vi "CPT32(Host).vi"() -> ()   [LabVIEW 2021]
uses:
  Control 1.ctl
  CPTLOCKIN/Control 2.ctl
  <vilib>/FPGAPlugInAG/PCIe-7857/niLvFpga_Open_PCIe-7857.vi
  <vilib>/rvi/interface/common/dynamic/niFpgaDynamicAddResources.vi
  <vilib>/Utility/error.llb/Error Cluster From Error Code.vi
  <vilib>/rvi/errors/niLvFpgaAdjustHostInterfaceError.vi
  <vilib>/FPGAPlugInAG/Dynamic/niLvFpga_Close_Dynamic.vi
  <vilib>/rvi/interface/nirviOpenFPGA/nirviOpenFPGA.xnode
  FPGA Bitfiles/lvfpga32_FPGATarget_CPT32PulseGen3(F_lvzEpAMTsdg.lvbitx
  FPGA Target/CPT32 Pulse Gen 3 (FPGA).vi
  <vilib>/rvi/interface/nirviReadWriteControl/nirviReadWriteControl.xnode
  <vilib>/rvi/interface/nirviCloseFPGA/nirviCloseFPGA.xnode
  <vilib>/rvi/interface/Simulation/niFpgaSimulationCallBeginRW.vi
  NiFpgaLv.dll
panel:
  in  "Tab Control":enum32{"数字与模拟信号控制"}(tab)
  in  "DO 0-7（ms）":T3={"DO 0"=[10.0, 0.0, 0.0, 0.0, 0.0, 0.0, 0.0, 0.0, 0.0, 0.0, 0.0, 0.0, 0.0, 0.0, 0.0, 0.0], "DO 1"=[-106.0, 0.2998046875, -20.0, 0.009765625, 0.0, 0.0, 0.0, 0.0, 0.0, 0.0, 0.0, 0.0, 0.0, 0.0, 0.0, 0.0, 0.0, 0.0, 0.0, 0.0, 0.0, 0.0, 0.0, 0.0, 0.0, 0.0, 0.0, 0.0, 0.0, 0.0, 0.0, 0.0], "DO 2"=[100.0, 5.0, 0.0, 0.0, 0.0, 0.0, 0.0, 0.0, 0.0, 0.0, 0.0, 0.0, 0.0, 0.0, 0.0, 0.0], "DO 3"=[100.0, 5.0, 0.0, 0.0, 0.0, 0.0, 0.0, 0.0, 0.0, 0.0, 0.0, 0.0, 0.0, 0.0, 0.0, 0.0], "DO 4"=[-100.0, 0.099609375, -27.0, 0.099609375, 0.0, 0.0, 0.0, 0.0, 0.0, 0.0, 0.0, 0.0, 0.0, 0.0, 0.0, 0.0, 0.0, 0.0, 0.0, 0.0, 0.0, 0.0, 0.0, 0.0, 0.0, 0.0, 0.0, 0.0, 0.0, 0.0, 0.0, 0.0], "DO 5"=[-106.0, 3.0, 0.0, 0.0, 0.0, 0.0, 0.0, 0.0, 0.0, 0.0, 0.0, 0.0, 0.0, 0.0, 0.0, 0.0, 0.0, 0.0, 0.0, 0.0, 0.0, 0.0, 0.0, 0.0, 0.0, 0.0, 0.0, 0.0, 0.0, 0.0, 0.0, 0.0], "DO 6"=[-105.0, 0.099609375, -27.0, 0.099609375, 0.0, 0.0, 0.0, 0.0, 0.0, 0.0, 0.0, 0.0, 0.0, 0.0, 0.0, 0.0, 0.0, 0.0, 0.0, 0.0, 0.0, 0.0, 0.0, 0.0, 0.0, 0.0, 0.0, 0.0, 0.0, 0.0, 0.0, 0.0], "DO 7"=[0.0, 0.0, 0.0, 0.0, 0.0, 0.0, 0.0, 0.0, 0.0, 0.0, 0.0, 0.0, 0.0, 0.0, 0.0, 0.0, 0.0, 0.0, 0.0, 0.0, 0.0, 0.0, 0.0, 0.0, 0.0, 0.0, 0.0, 0.0, 0.0, 0.0, 0.0, 0.0]} {"DO 7" format="%#.3g"; "DO 6" format="%#.3g"; "DO 5" format="%#.3g"; "DO 4" format="%#.3g"; "DO 3" format="%#.3g"; "DO 2" format="%#.3g"; "DO 1" format="%#.3g"; "DO 0" format="%#.3g"}
  in  "总时间 (ms)":fxp<+,32,16>=135.0
  in  "Quit":bool
  in  "Start":bool
  in  "Stop":bool
  out "运行状态-LED":bool caption="运行状态"
  out "已运行时间 (s)":dbl
  in  "AO 0":T4={"Time 0 (ms)"=[50.0, 5.0, 1.0, 0.0, 0.0, 0.0, 0.0, 0.0, 0.0, 0.0, 0.0, 0.0, 0.0, 0.0, 0.0, 0.0], "Voltage 0 (V)"=[0.29999999701976776, 0.2800000011920929, 0.0, 0.0, 0.0, 0.0, 0.0, 0.0, 0.0, 0.0, 0.0, 0.0, 0.0, 0.0, 0.0, 0.0]} {"Voltage 0 (V)" format="%#.6g"; "Time 0 (ms)" format="%#.3g"}
  in  "AO 1":T5={"Time 1 (ms)"=[25.0, 25.0, 25.0, 25.0, 0.0, 0.0, 0.0, 0.0, 0.0, 0.0, 0.0, 0.0, 0.0, 0.0, 0.0, 0.0], "Voltage 1 (V)"=[1.0, 2.0, 3.0, 4.0, 0.0, 0.0, 0.0, 0.0, 0.0, 0.0, 0.0, 0.0, 0.0, 0.0, 0.0, 0.0]} {"Voltage 1 (V)" format="%#.6g"; "Time 1 (ms)" format="%#.3g"}
  in  "AO 2":T6={"Time 2 (ms)"=[0.0, 0.0, 0.0, 0.0], "Voltage 2 (V)"=[0.0, 0.0, 0.0, 0.0]} {"Voltage 2 (V)" format="%#.6g"; "Time 2 (ms)" format="%#.3g"}
  in  "AO 3":T7={"Time 3 (ms)"=[0.0, 0.0, 0.0, 0.0], "Voltage 3 (V)"=[0.0, 0.0, 0.0, 0.0]} {"Voltage 3 (V)" format="%#.6g"; "Time 3 (ms)" format="%#.3g"}
  in  "读取总控件":bool
  in  "保存总控件":bool
  # "中山大学 量子工程与精密测量实验室 CPT信号控制系统"
  # "操作说明：\n1、数字信号控制为DO，输入数据正数为高电平，负数为低电平，单位ms，DO 0,2,3,4,6,7时间段上限为16段,DO 1,5上限为32段；\n2、模拟信号控制为AO，时间栏输入控制时间，电压栏输入对应时间内电压大小，范围（-10V~10V）；\n3、先停止循环再退出程序，否则会持续输出；\n3、定义时间不能超过总时间，否则周期由最长总定义时间决定；\n4、fixed-point 数据格式：时间 word 21 int 11（max=1024,delta~=0.001）；电压 word 32 int 6（max=32, delta~=1e-8）；"
  # "AO reset"
  # "CPT/Probe"
  # "780"
  # "795"
  # "MOT-B"
  # "Trigger"
  # "Bias-B"
  # "CCD"
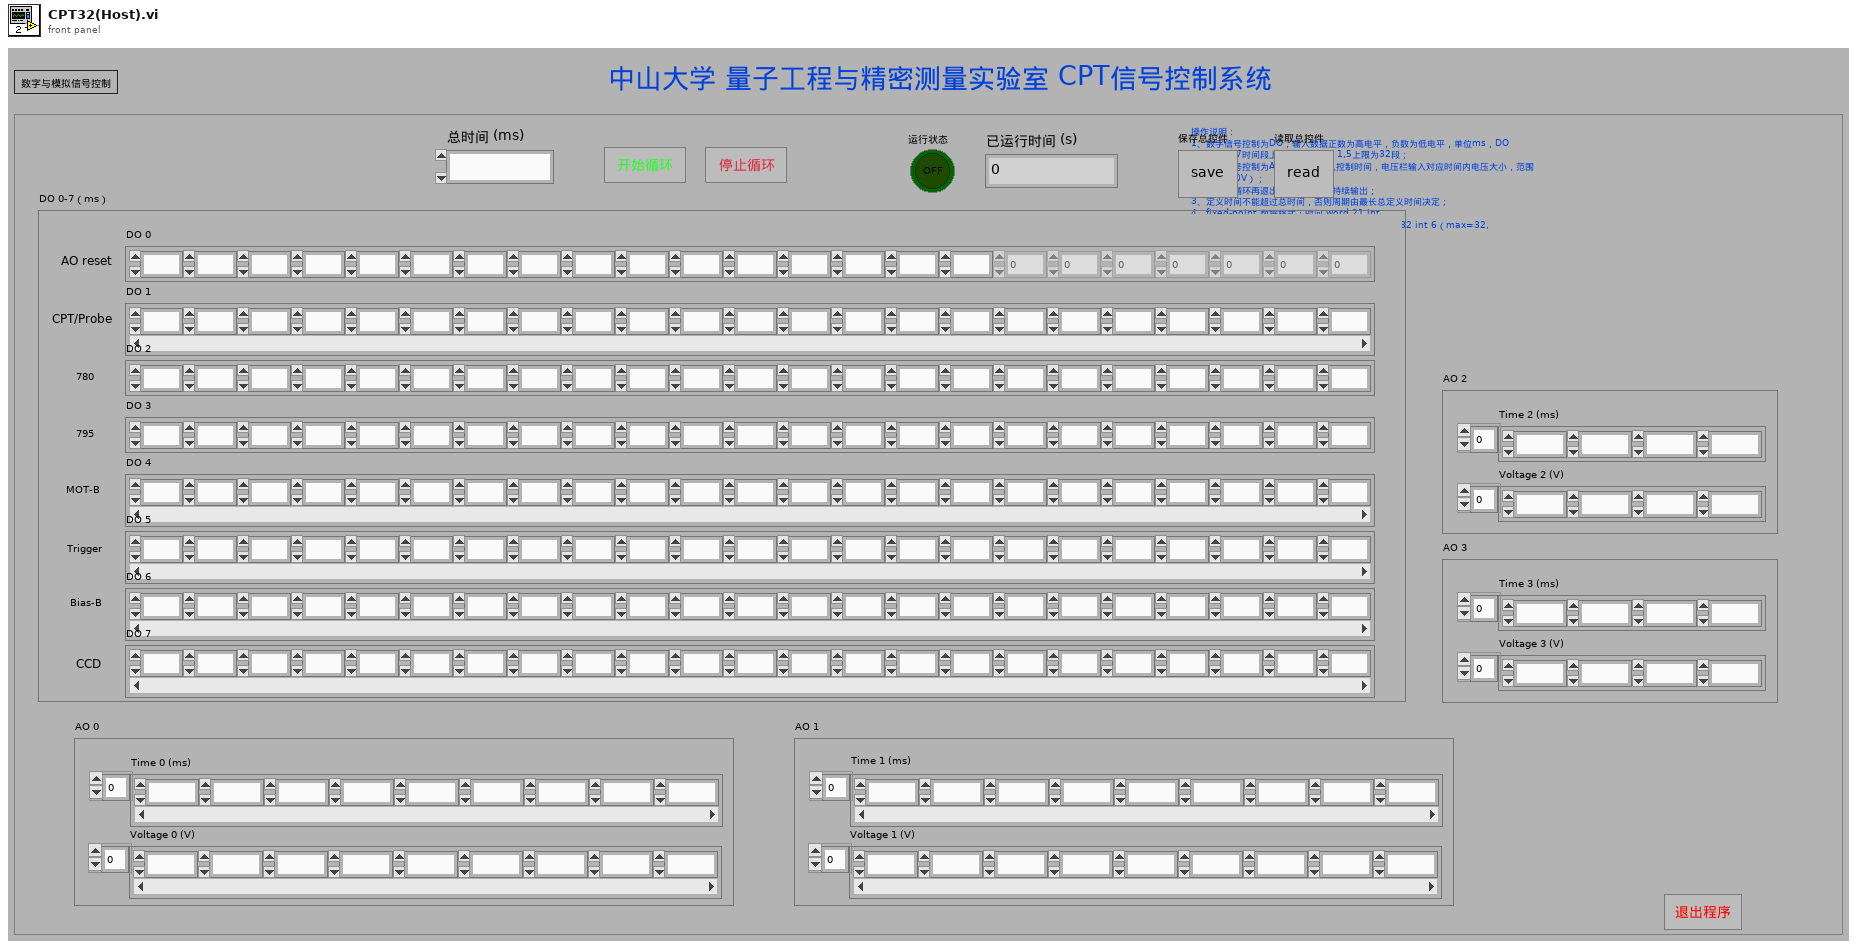
[diagram p1: front panel]
types:
  T1 = typedef "Control 1.ctl" = fxp<+/-,21,11>
  T2 = typedef "Control 2.ctl" = fxp<+/-,21,11>[]
  T3 = cluster{"DO 0":fxp<+/-,21,11>[], "DO 1":T1[], "DO 2":fxp<+/-,21,11>[], "DO 3":fxp<+/-,21,11>[], "DO 4":fxp<+/-,21,11>[], "DO 5":fxp<+/-,21,11>[], "DO 6":T2, "DO 7":fxp<+/-,21,11>[]}
  T4 = cluster{"Time 0 (ms)":fxp<+/-,21,11>[], "Voltage 0 (V)":fxp<+/-,32,6>[]}
  T5 = cluster{"Time 1 (ms)":fxp<+/-,21,11>[], "Voltage 1 (V)":fxp<+/-,32,6>[]}
  T6 = cluster{"Time 2 (ms)":fxp<+/-,21,11>[], "Voltage 2 (V)":fxp<+/-,32,6>[]}
  T7 = cluster{"Time 3 (ms)":fxp<+/-,21,11>[], "Voltage 3 (V)":fxp<+/-,32,6>[]}
  T8 = cluster{"总时间 (ms)":dbl, "DO 0-7":cluster{"Port 0 Channel 1":dbl[], "Port 0 Channel 2":dbl[], "Port 0 Channel 3":dbl[], "Port 0 Channel 4":dbl[], "Port 0 Channel 5":dbl[], "Port 0 Channel 6":dbl[], "Port 0 Channel 7":dbl[], "Port 0 Channel 0":dbl[]}, "AO 0":cluster{"Port 0 Channel 1":dbl[], "Port 0 Channel 2":dbl[]}, "AO 1":cluster{"Port 0 Channel 1":dbl[], "Port 0 Channel 2":dbl[]}, "AO 2":cluster{"Port 0 Channel 1":dbl[], "Port 0 Channel 2":dbl[]}, "AO 3":cluster{"Port 0 Channel 1":dbl[], "Port 0 Channel 2":dbl[]}}
  T9 = cluster{"Port 0 Channel 1":dbl[], "Port 0 Channel 2":dbl[], "Port 0 Channel 3":dbl[], "Port 0 Channel 4":dbl[], "Port 0 Channel 5":dbl[], "Port 0 Channel 6":dbl[], "Port 0 Channel 7":dbl[], "Port 0 Channel 0":dbl[]}
  T10 = cluster{"Port 0 Channel 1":dbl[], "Port 0 Channel 2":dbl[]}
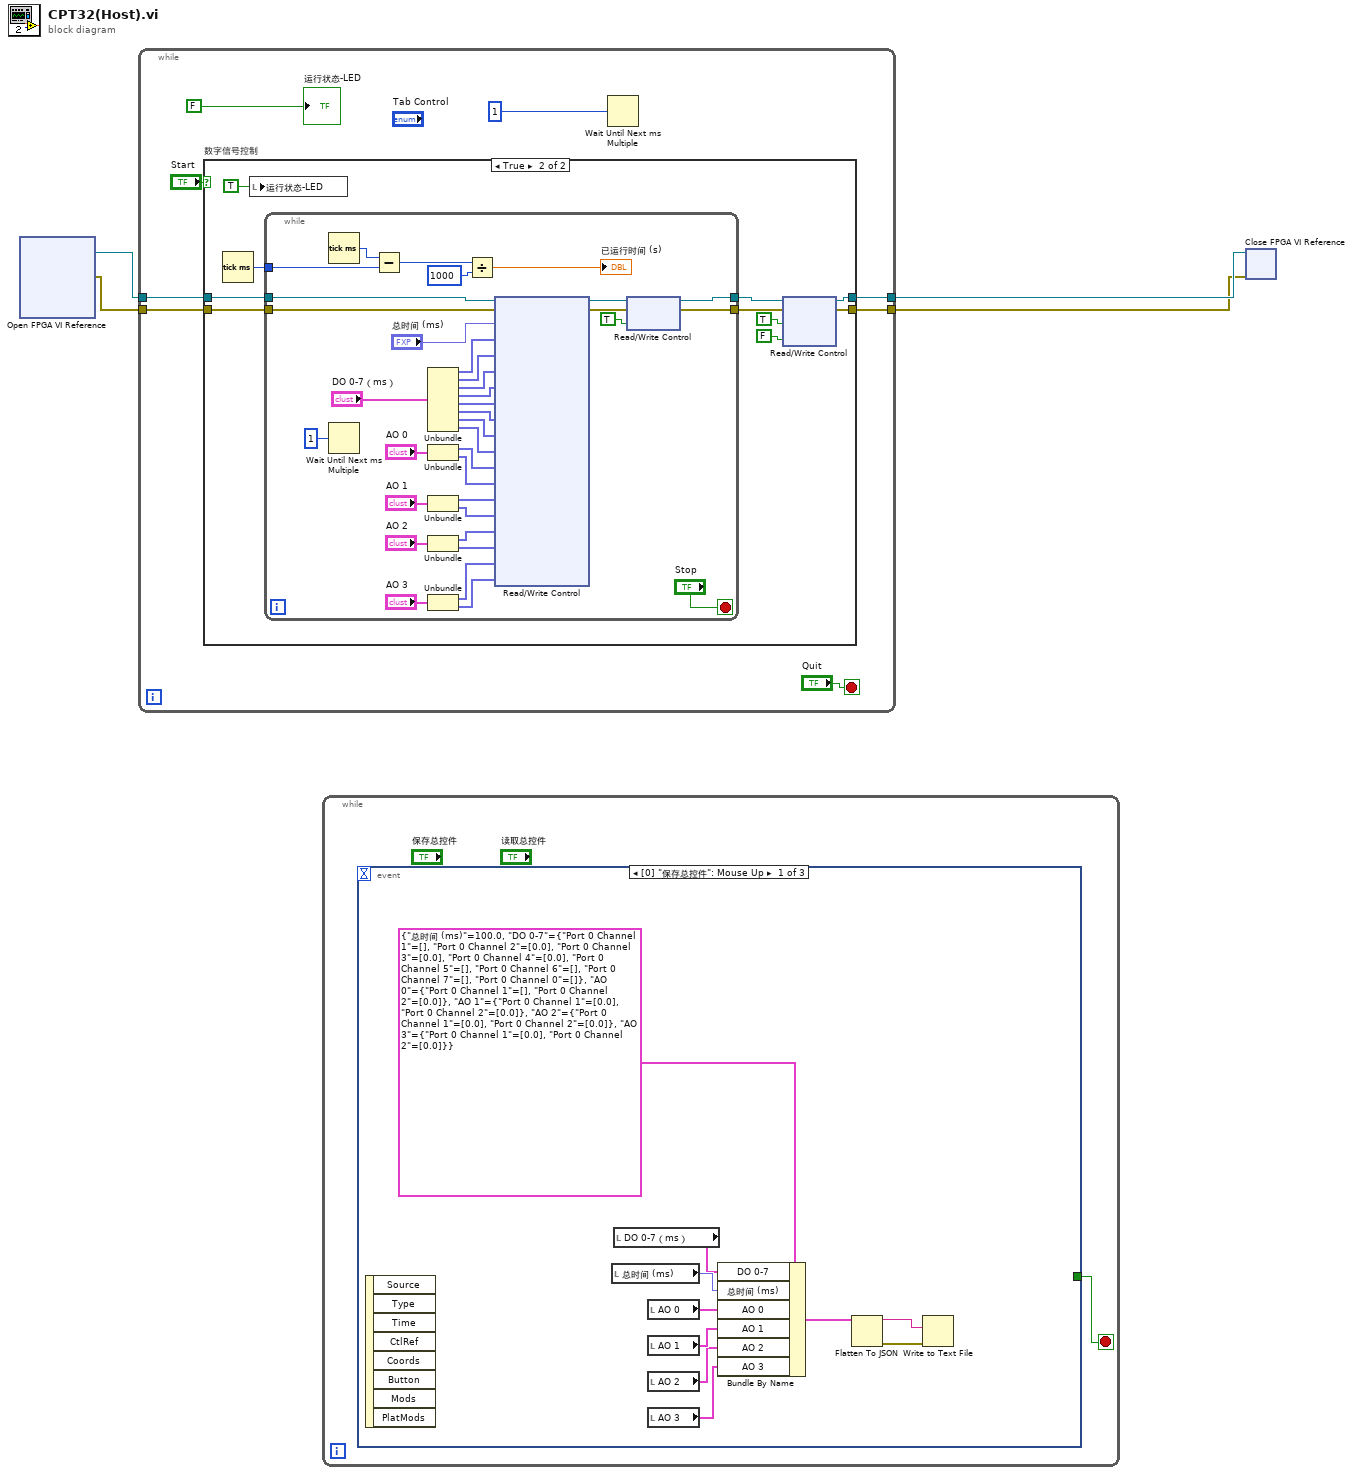
[diagram p0: block diagram]
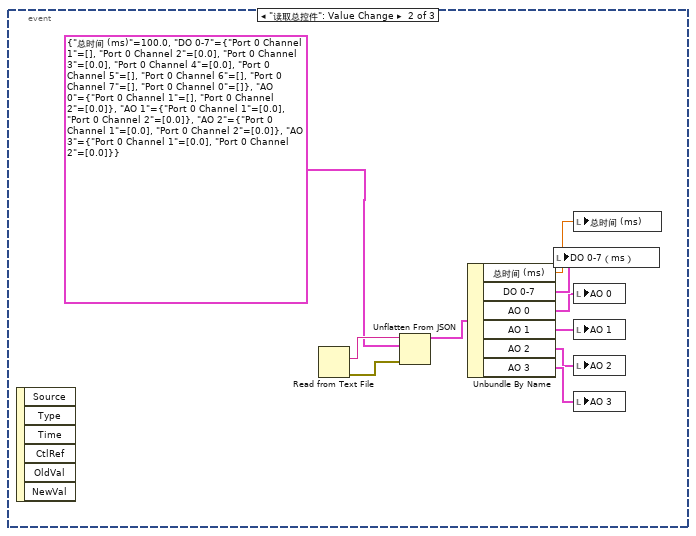
[diagram p2: hidden frame]
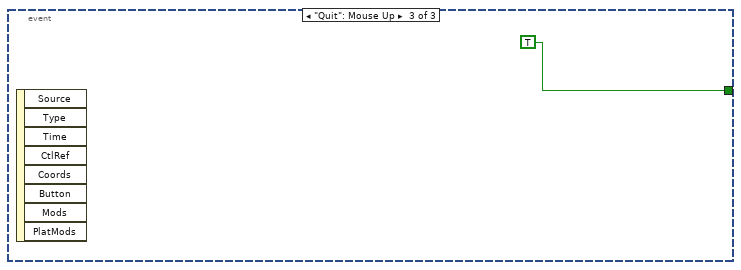
[diagram p3: hidden frame]
diagram:
  n1 = xnode "Open FPGA VI Reference"() -> ("FPGA VI Reference Out"=w2:refnum<k20>, "error out"=w1:errorcluster)  [unwired: 2 in]
  n2 = while {
    tunnel: w2 -> [w7]
    tunnel: w1 -> [w6]
    tunnel: [w10] -> w4
    tunnel: [w9] -> w3
    stop <- "Quit" stop-if-true
    n3 = case "数字信号控制" shown="True" "Start" {
      tunnel: w7 -> [w14 w16]
      tunnel: w6 -> [w13 w15]
      tunnel: [w14 w24] -> w10
      tunnel: [w13 w23] -> w9
      frame False {
      }
      frame True {
        n4 = Tick Count (ms)() -> (millisecond timer value=w21:u32)
        n5 = local write "运行状态-LED"(TRUE ("运行状态-LED")) -> ()
        n6 = while {
          tunnel: w21 -> [w54]
          tunnel: [w53] -> w18
          tunnel: [w52] -> w17
          tunnel: w16 -> [w28]
          tunnel: w15 -> [w27]
          stop <- "Stop" stop-if-true
          n7 = Tick Count (ms)() -> (millisecond timer value=w58:u32)
          n8 = Wait Until Next ms Multiple(millisecond multiple=u32 1) -> ()  [unwired: 1 out]
          n9 = Subtract(x=w58, y=w54) -> (x-y=w57:u32)
          n10 = Unbundle("DO 0-7（ms）") -> ("DO 0"=w46:fxp<+/-,21,11>[], "DO 1"=w45:T1[], "DO 2"=w44:fxp<+/-,21,11>[], "DO 3"=w43:fxp<+/-,21,11>[], "DO 4"=w42:fxp<+/-,21,11>[], "DO 5"=w41:fxp<+/-,21,11>[], "DO 6"=w40:T2, "DO 7"=w39:fxp<+/-,21,11>[])
          n11 = Unbundle("AO 0") -> ("Time 0 (ms)"=w34:fxp<+/-,21,11>[], "Voltage 0 (V)"=w33:fxp<+/-,32,6>[])
          n12 = Unbundle("AO 1") -> ("Time 1 (ms)"=w32:fxp<+/-,21,11>[], "Voltage 1 (V)"=w31:fxp<+/-,32,6>[])
          n13 = Unbundle("AO 2") -> ("Time 2 (ms)"=w30:fxp<+/-,21,11>[], "Voltage 2 (V)"=w29:fxp<+/-,32,6>[])
          n14 = Unbundle("AO 3") -> ("Time 3 (ms)"=w49:fxp<+/-,21,11>[], "Voltage 3 (V)"=w48:fxp<+/-,32,6>[])
          n15 = Divide(x=w57, y=u32 1000) -> (x/y=→"已运行时间 (s)":dbl)
          n16 = xnode "Read/Write Control"("FPGA VI Reference In"=w28, "error in"=w27, "Period (ms)"="总时间 (ms)", "DO 0"=w46, "DO 1"=w45, "DO 2"=w44, "DO 3"=w43, "DO 4"=w42, "DO 5"=w41, "DO 6"=w40, "DO 7"=w39, "AO 0 time"=w34, "AO 0 voltage"=w33, "AO 1 time"=w32, "AO 1 voltage"=w31, "AO 2 time"=w30, "AO 2 voltage"=w29, "AO 3 time"=w49, "AO 3 voltage"=w48) -> ("FPGA VI Reference Out"=w26:refnum<k20>, "error out"=w25:errorcluster)
          n17 = xnode "Read/Write Control"("FPGA VI Reference In"=w26, "error in"=w25, "Start"=TRUE) -> ("FPGA VI Reference Out"=w53:refnum<k20>, "error out"=w52:errorcluster)
        }
        n18 = xnode "Read/Write Control"("FPGA VI Reference In"=w18, "error in"=w17, "Stop"=TRUE, "Start"=FALSE) -> ("FPGA VI Reference Out"=w24:refnum<k20>, "error out"=w23:errorcluster)
      }
    }
    n19 = Wait Until Next ms Multiple(millisecond multiple=u32 1) -> ()  [unwired: 1 out]
    "运行状态-LED" <- FALSE
  }
  n20 = while {
    stop <- w61 stop-if-true
    n21 = event shown="[0] \"保存总控件\": Mouse Up" {
      selector: _ -> [_ _ _]
      dyn-events: _ -> [_ _ _]
      timeout: _ -> [_ _ _]
      tunnel: [_ _ TRUE] -> w61
      event "保存总控件": Mouse Up {
        n22 = event-data() -> ()  [unwired: 1 in, 8 out]
        n23 = local read "总时间 (ms)"() -> (w71:fxp<+,32,16>)
        n24 = local read "DO 0-7（ms）"() -> (w66:T3)
        n25 = local read "AO 0"() -> (w70:T4)
        n26 = local read "AO 1"() -> (w65:T5)
        n27 = local read "AO 2"() -> (w64:T6)
        n28 = local read "AO 3"() -> (w63:T7)
        n29 = Bundle By Name(cluster=T8 {"总时间 (ms)"=100.0, "DO 0-7"={"Port 0 Channel 1"=[], "Port 0 Channel 2"=[0.0], "Port 0 Channel 3"=[0.0], "Port 0 Channel 4"=[0.0], "Port 0 Channel 5"=[], "Port 0 Channel 6"=[], "Port 0 Channel 7"=[], "Port 0 Channel 0"=[]}, "AO 0"={"Port 0 Channel 1"=[], "Port 0 Channel 2"=[0.0]}, "AO 1"={"Port 0 Channel 1"=[0.0], "Port 0 Channel 2"=[0.0]}, "AO 2"={"Port 0 Channel 1"=[0.0], "Port 0 Channel 2"=[0.0]}, "AO 3"={"Port 0 Channel 1"=[0.0], "Port 0 Channel 2"=[0.0]}}, "DO 0-7"=w66, "总时间 (ms)"=w71, "AO 0"=w70, "AO 1"=w65, "AO 2"=w64, "AO 3"=w63) -> (w69:T8)
        n30 = Flatten To JSON(anything=w69) -> (JSON string=w67:string, 11:w68:errorcluster)  [unwired: 2 in]
        n31 = Write to Text File(text=w67, error in=w68) -> ()  [unwired: 2 in, 3 out]
      }
      event "读取总控件": Value Change {
        n32 = event-data() -> ()  [unwired: 1 in, 6 out]
        n33 = Read from Text File() -> (text=w81:string, error out=w80:errorcluster)  [unwired: 4 in, 2 out]
        n34 = Unflatten From JSON(JSON string=w81, type and defaults=T8 {"总时间 (ms)"=100.0, "DO 0-7"={"Port 0 Channel 1"=[], "Port 0 Channel 2"=[0.0], "Port 0 Channel 3"=[0.0], "Port 0 Channel 4"=[0.0], "Port 0 Channel 5"=[], "Port 0 Channel 6"=[], "Port 0 Channel 7"=[], "Port 0 Channel 0"=[]}, "AO 0"={"Port 0 Channel 1"=[], "Port 0 Channel 2"=[0.0]}, "AO 1"={"Port 0 Channel 1"=[0.0], "Port 0 Channel 2"=[0.0]}, "AO 2"={"Port 0 Channel 1"=[0.0], "Port 0 Channel 2"=[0.0]}, "AO 3"={"Port 0 Channel 1"=[0.0], "Port 0 Channel 2"=[0.0]}}, error in (no error)=w80) -> (value=w79:T8)  [unwired: 4 in, 1 out]
        n35 = Unbundle By Name(w79) -> ("总时间 (ms)"=w77:dbl, "DO 0-7"=w78:T9, "AO 0"=w73:T10, "AO 1"=w74:T10, "AO 2"=w75:T10, "AO 3"=w76:T10)
        n36 = local write "DO 0-7（ms）"(w78) -> ()
        n37 = local write "总时间 (ms)"(w77) -> ()
        n38 = local write "AO 0"(w73) -> ()
        n39 = local write "AO 1"(w74) -> ()
        n40 = local write "AO 2"(w75) -> ()
        n41 = local write "AO 3"(w76) -> ()
      }
      event "Quit": Mouse Up {
        n42 = event-data() -> ()  [unwired: 1 in, 8 out]
      }
    }
  }
  n43 = xnode "Close FPGA VI Reference"("FPGA VI Reference In"=w4, "error in"=w3) -> ()  [unwired: 1 out]
